vi "主动发送数据生成Condition(子VI).vi"(8 "数据发送协议":enum16{"2005-212协议", "2017-212协议"}(ring)=enum."2017-212协议", 9 "database":string, 10 "Label.Text":string, 11 "数值":i32) -> (2 "columns":string[](array[string])=["时间", "测量模式", "数据类型", "检测值", "单位", "数据标识"], 3 "CONDITION":string)   [LabVIEW 2016, in "数据传输系统.lvlib"]
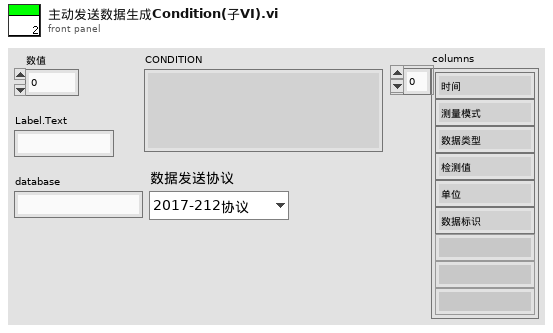
[diagram p1: front panel]
types:
  T1 = typedef "LVDateTimeRec.ctl" = cluster{"秒数的小数部分":dbl, "秒":i32, "分":i32, "时":i32, "日":i32, "月":i32, "年":i32, "天数（周）":i32, "天数（年）":i32, "DST":i32}
  T2 = cluster{"time1":string, "time2":string, "time3":string, "time4":string, "time5":string, "time6":string, "time7":string, "time8":string, "time9":string, "time10":string, "time11":string, "time12":string, "time13":string, "time14":string, "time15":string, "time16":string, "time17":string, "time18":string, "time19":string, "time20":string, "time21":string, "time22":string, "time23":string, "time24":string, "time25":string, "time26":string, "time27":string, "time28":string, "time29":string, "time30":string, "time31":string}
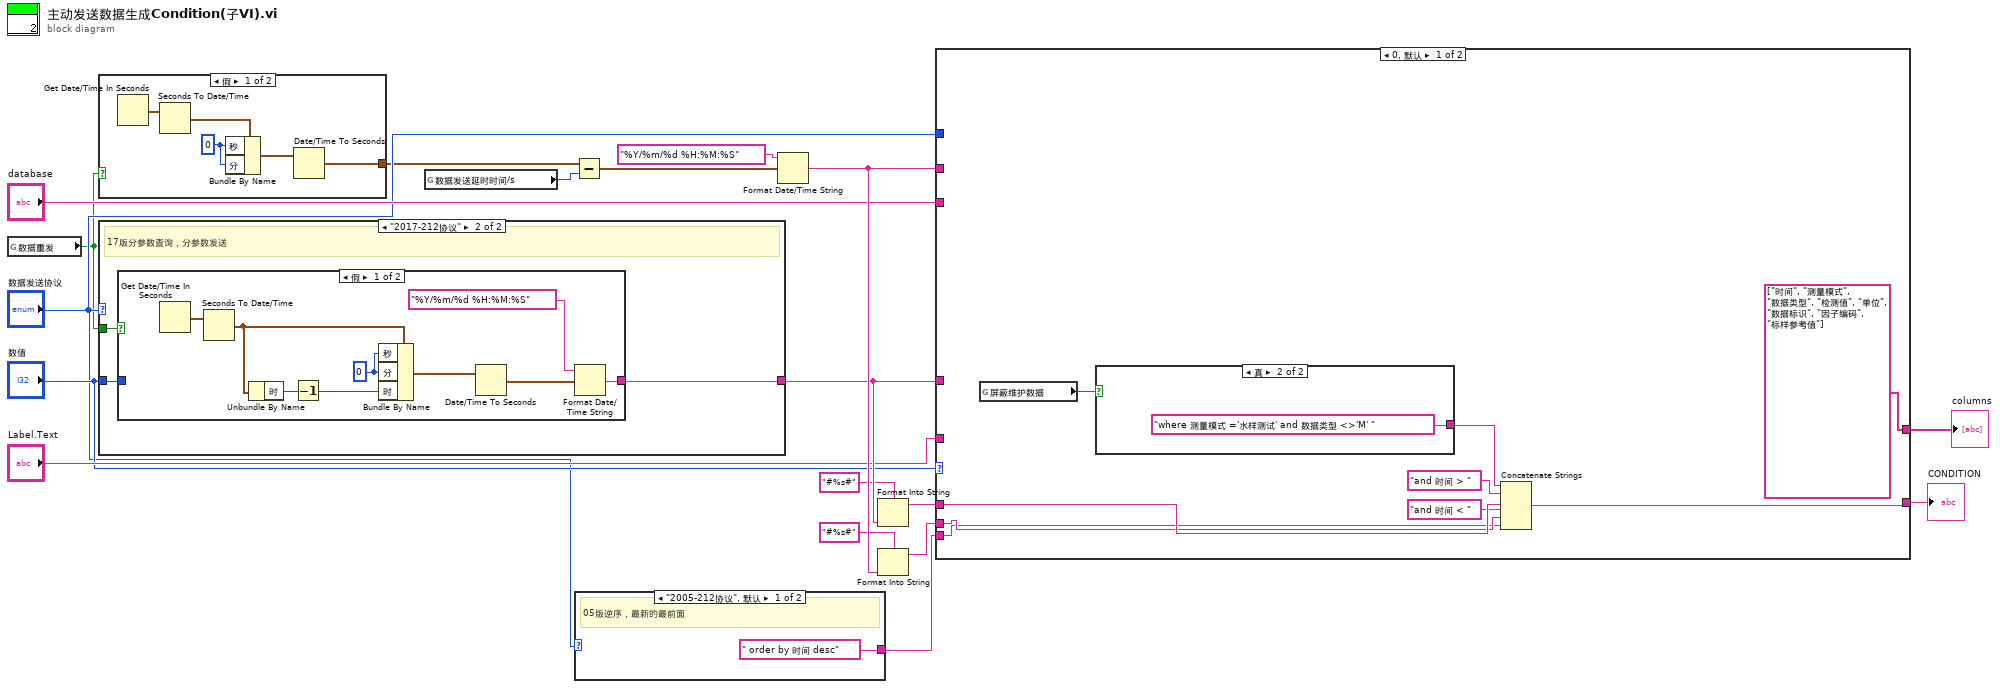
[diagram p0: block diagram]
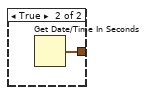
[diagram p2: hidden frame]
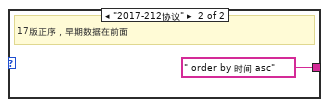
[diagram p3: hidden frame]
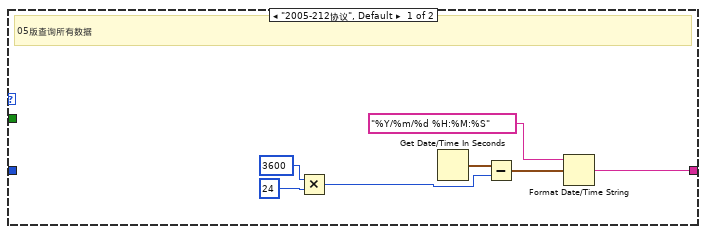
[diagram p4: hidden frame]
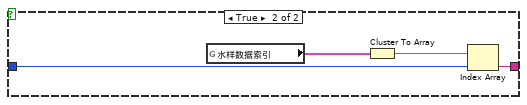
[diagram p5: hidden frame]
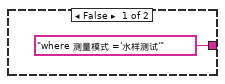
[diagram p6: hidden frame]
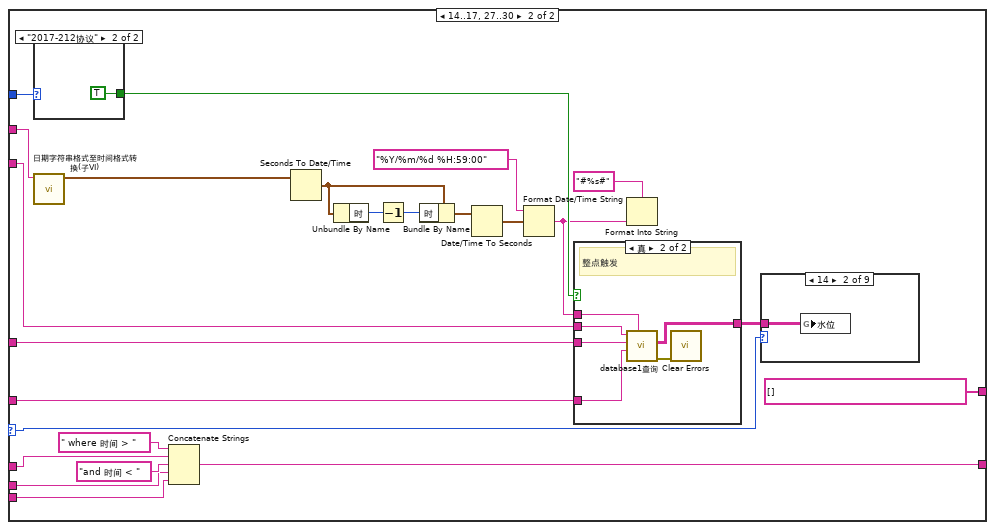
[diagram p7: hidden frame]
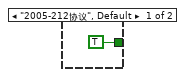
[diagram p8: hidden frame]
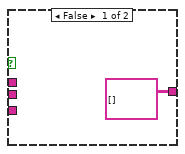
[diagram p9: hidden frame]
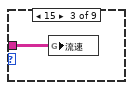
[diagram p11: hidden frame]
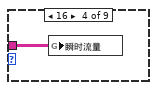
[diagram p12: hidden frame]
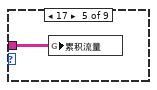
[diagram p13: hidden frame]
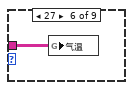
[diagram p14: hidden frame]
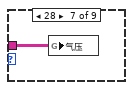
[diagram p15: hidden frame]
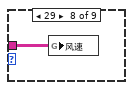
[diagram p16: hidden frame]
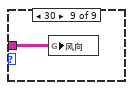
[diagram p17: hidden frame]
diagram:
  n1 = global read "断电保存全局.vi" "数据重发"() -> (w1:bool)
  n2 = case shown="假" w1 {
    tunnel: [w19 w24] -> w3
    frame False {
      w23 = 0 ("秒")
      n3 = Get Date/Time In Seconds() -> (seconds since 1Jan1904=w20:timestamp)
      n4 = Seconds To Date/Time(time stamp (now)=w20) -> (date time rec=w21:T1)  [unwired: 1 in]
      n5 = Bundle By Name(cluster=w21, "秒"=w23, "分"=w23) -> (w22:T1)
      n6 = Date/Time To Seconds(2:w22) -> (0:w19:timestamp)  [unwired: 1 in]
    }
    frame True {
      n7 = Get Date/Time In Seconds() -> (seconds since 1Jan1904=w24:timestamp)
    }
  }
  n8 = case shown="\"2017-212协议\"" "数据发送协议" {
    tunnel: [w30 w33] -> w17
    tunnel: "数值" -> [_ w34]
    tunnel: w1 -> [_ w32]
    frame "2005-212协议", Default {
      # "05版查询所有数据"
      n9 = Multiply(x=3600, y=24) -> (x*y=w25:i32)
      n10 = Get Date/Time In Seconds() -> (seconds since 1Jan1904=w29:timestamp)
      n11 = Subtract(x=w29, y=w25) -> (x-y=w28:timestamp)
      n12 = Format Date/Time String(time format string (%c)="%Y/%m/%d %H:%M:%S" ("时间格式字符串(%c)"), seconds (now)=w28) -> (date/time string=w30:string)  [unwired: 1 in]
    }
    frame "2017-212协议" {
      # "17版分参数查询，分参数发送"
      n13 = case shown="假" w32 {
        tunnel: w34 -> [_ w45]
        tunnel: [w35 w44] -> w33
        frame False {
          w38 = 0 ("秒")
          n14 = Get Date/Time In Seconds() -> (seconds since 1Jan1904=w36:timestamp)
          n15 = Seconds To Date/Time(time stamp (now)=w36) -> (date time rec=w39:T1)  [unwired: 1 in]
          n16 = Unbundle By Name(w39) -> ("时"=w40:i32)
          n17 = Decrement(x=w40) -> (x-1=w41:i32)
          n18 = Bundle By Name(cluster=w39, "秒"=w38, "分"=w38, "时"=w41) -> (w37:T1)
          n19 = Date/Time To Seconds(2:w37) -> (0:w43:timestamp)  [unwired: 1 in]
          n20 = Format Date/Time String(time format string (%c)="%Y/%m/%d %H:%M:%S" ("时间格式字符串(%c)"), seconds (now)=w43) -> (date/time string=w35:string)  [unwired: 1 in]
        }
        frame True {
          n21 = global read "全局 水样时间.vi" "水样数据索引"() -> (w46:T2)
          n22 = Cluster To Array(cluster=w46) -> (array=w47:string[])
          n23 = Index Array(array=w47, index=w45) -> (element=w44:string)
        }
      }
    }
  }
  n24 = global read "断电保存全局.vi" "数据发送延时时间/s"() -> (w4:i32)
  n25 = Subtract(x=w3, y=w4) -> (x-y=w2:timestamp)
  n26 = case shown="\"2005-212协议\", 默认" "数据发送协议" {
    tunnel: [" order by 时间 desc" ("字符串") " order by 时间 asc" ("字符串")] -> w7
    frame "2005-212协议", Default {
      # "05版逆序，最新的最前面"
    }
    frame "2017-212协议" {
      # "17版正序，早期数据在前面"
    }
  }
  n27 = Format Date/Time String(time format string (%c)="%Y/%m/%d %H:%M:%S" ("时间格式字符串(%c)"), seconds (now)=w2) -> (date/time string=w18:string)  [unwired: 1 in]
  n28 = Format Into String(format string="#%s#" ("初始字符串"), w17) -> (resulting string=w11:string)  [unwired: 2 in, 1 out]
  n29 = Format Into String(format string="#%s#" ("初始字符串"), w18) -> (resulting string=w13:string)  [unwired: 2 in, 1 out]
  n30 = case shown="0, 默认" "数值" {
    selector: "数值" -> [_ w77]
    tunnel: w11 -> [w58 w81]
    tunnel: [w57 w82] -> w12
    tunnel: w13 -> [w55 w62]
    tunnel: "database" -> [_ w80]
    tunnel: "Label.Text" -> [_ w79]
    tunnel: w17 -> [_ w61]
    tunnel: w18 -> [_ w65]
    tunnel: w7 -> [w53 w76]
    tunnel: [string[] ["时间", "测量模式", "数据类型", "检测值", "单位", "数据标识", "因子编码", "标样参考值"] ("columns") string[] [] ("columns")] -> w6
    tunnel: "数据发送协议" -> [_ w73]
    frame 0, Default {
      n31 = global read "断电保存全局.vi" "屏蔽维护数据"() -> (w51:bool)
      n32 = case shown="真" w51 {
        tunnel: ["where 测量模式 ='水样测试'" ("condition") "where 测量模式 ='水样测试' and 数据类型 <>'M' "] -> w50
        frame False {
        }
        frame True {
        }
      }
      n33 = Concatenate Strings(w50, "and 时间 > ", w58, "and 时间 < " ("字符串"), w55, w53) -> (w57:string)
    }
    frame 14..17, 27..30 {
      n34 = case shown="\"2017-212协议\"" w73 {
        tunnel: [TRUE TRUE] -> w75
        frame "2005-212协议", Default {
        }
        frame "2017-212协议" {
        }
      }
      n35 = call "日期字符串格式至时间格式转换(子VI).vi"("data[0]"=w65) -> ("time stamp"=w68:timestamp)  [unwired: 10 in]
      n36 = Concatenate Strings(" where 时间 > ", w81, "and 时间 < " ("字符串"), w62, w76) -> (w82:string)
      n37 = Seconds To Date/Time(time stamp (now)=w68) -> (date time rec=w70:T1)  [unwired: 1 in]
      n38 = Unbundle By Name(w70) -> ("时"=w71:i32)
      n39 = Decrement(x=w71) -> (x-1=w72:i32)
      n40 = Bundle By Name(cluster=w70, "时"=w72) -> (w69:T1)
      n41 = Date/Time To Seconds(2:w69) -> (0:w67:timestamp)  [unwired: 1 in]
      n42 = Format Date/Time String(time format string (%c)="%Y/%m/%d %H:59:00" ("时间格式字符串(%c)"), seconds (now)=w67) -> (date/time string=w63:string)  [unwired: 1 in]
      n43 = case shown="真" w75 {
        tunnel: w80 -> [_ w93]
        tunnel: w79 -> [_ w92]
        tunnel: [string[][] [] ("data") w91] -> w78
        tunnel: w63 -> [_ w90]
        tunnel: w61 -> [_ w88]
        frame False {
        }
        frame True {
          # "整点触发"
          n44 = call "database1查询.vi"("时间2"=w90, "table"=w92, "时间1"=w88, "database"=w93) -> ("error out"=w89:errorcluster, "data"=w91:string[][])  [unwired: 4 in, 1 out]
          n45 = call <vilib>:"Clear Errors.vi"("error in (no error)"=w89) -> ()  [unwired: 5 in, 2 out]
        }
      }
      n46 = Format Into String(format string="#%s#" ("初始字符串"), w63) -> ()  [unwired: 2 in, 2 out]
      n47 = case shown="14" w77 {
        tunnel: w78 -> [_ w94 w95 w96 w97 w98 w99 w100 w101]
        frame 0, Default {
        }
        frame 14 {
          n48 = global write "全局 所有参数.vi" "水位"(w94) -> ()
        }
        frame 15 {
          n49 = global write "全局 所有参数.vi" "流速"(w95) -> ()
        }
        frame 16 {
          n50 = global write "全局 所有参数.vi" "瞬时流量"(w96) -> ()
        }
        frame 17 {
          n51 = global write "全局 所有参数.vi" "累积流量"(w97) -> ()
        }
        frame 27 {
          n52 = global write "全局 所有参数.vi" "气温"(w98) -> ()
        }
        frame 28 {
          n53 = global write "全局 所有参数.vi" "气压"(w99) -> ()
        }
        frame 29 {
          n54 = global write "全局 所有参数.vi" "风速"(w100) -> ()
        }
        frame 30 {
          n55 = global write "全局 所有参数.vi" "风向"(w101) -> ()
        }
      }
    }
  }
  "CONDITION" <- w12
  "columns" <- w6
